vi "load config data.vi"(8 "error in (no error)":errorcluster, 11 "Imaq Camera in":refnum<class "Imaq Camera.lvclass">) -> (0 "error out":errorcluster, 3 "Imaq Camera out":refnum<class "Imaq Camera.lvclass">)   [LabVIEW 2022 SP3, in "Imaq Camera.lvclass"]
uses:
  Imaq Camera.lvclass
  C:/XY Stage/XY Stage/Framework/Base/Base.lvclass
  XY Stage/Framework/Base/Base.lvclass/Base.ctl
  Imaq Camera.lvclass/Imaq Camera.ctl
  243eee28-49f0-474d-8ecb-0c8253db1a59.vi
  XY Stage/Framework/Base/Accessors/Read Config Path.vi
  XY Stage/Framework/Base/Accessors/Read Section.vi
  <vilib>/Utility/config.llb/Open Config Data.vi
  <userlib>/_OpenG.lib/variantconfig/variantconfig.llb/Read Section Cluster__ogtk.vi
  <vilib>/Utility/config.llb/Close Config Data.vi
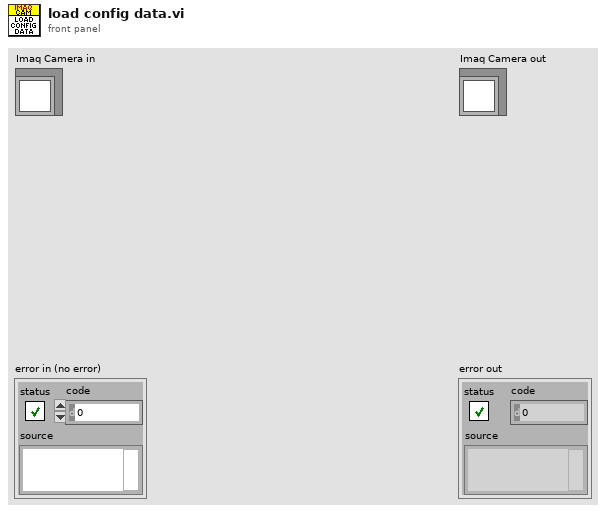
[diagram p1: front panel]
types:
  T1 = typedef "Imaq Camera.lvclass/Settings.ctl" = cluster{"Camera Name":string}
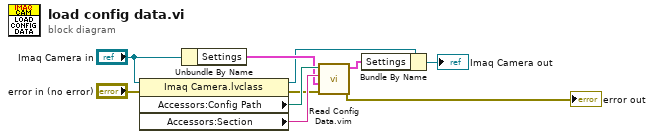
[diagram p0: block diagram]
diagram:
  n1 = property class="Imaq Camera.lvclass"(reference="Imaq Camera in", error in="error in (no error)") -> (reference out=w5:refnum<class "Imaq Camera.lvclass">, error out=w2:errorcluster, "Accessors:Config Path"=w10:path, "Accessors:Section"=w9:string)
  n2 = Unbundle By Name("Imaq Camera in") -> ("Settings"=w6:T1)
  n3 = call "Read Config Data.vim"("error in (no error)"=w2, "Section Formatted Cluster Type"=w6, "Section"=w9, "Config Path"=w10) -> ("error out"=→"error out":errorcluster, "Section Formatted Cluster Type 2"=w4:T1)  [unwired: 6 in]
  n4 = Bundle By Name(cluster=w5, "Settings"=w4) -> (→"Imaq Camera out":refnum<class "Imaq Camera.lvclass">)
